vi "Get Segment Limits.vi"(8 "error in (no error)":errorcluster, 10 "segmentIdxIn":i32, 11 "TreeNode in":refnum<class "TreeNode.lvclass">) -> (0 "error out":errorcluster, 1 "End Data out":refnum<class "Data.lvclass">, 2 "Start Data out":refnum<class "Data.lvclass">, 3 "TreeNode out":refnum<class "TreeNode.lvclass">)   [LabVIEW 2012, in "MDSplus.lvlib" / "TreeNode.lvclass"]
uses:
  <vilib>/MDSplus/Classes/Data_Class/TreeNode_Class/TreeNode.lvclass
  <vilib>/MDSplus/Classes/Data_Class/Data.lvclass
  MDSobjectsLVShr.dll
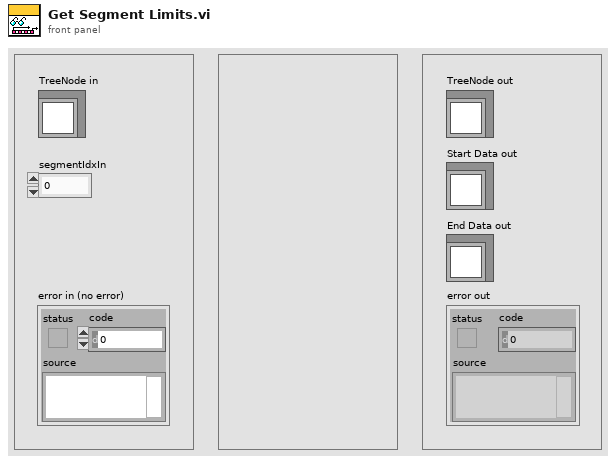
[diagram p1: front panel]
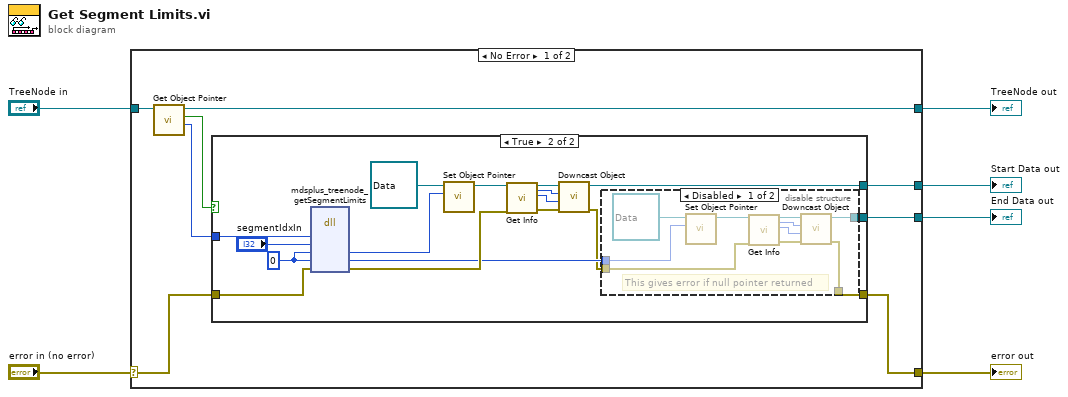
[diagram p0: block diagram]
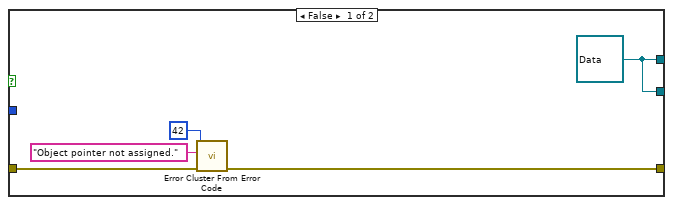
[diagram p2: hidden frame]
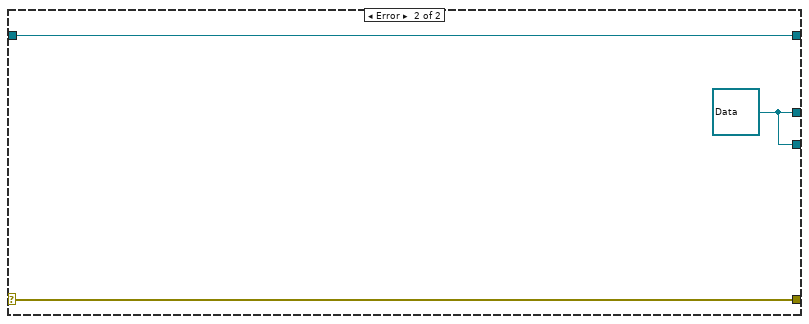
[diagram p4: hidden frame]
diagram:
  n1 = case shown="No Error" "error in (no error)" {
    selector: "error in (no error)" -> [w10 w50]
    tunnel: [w7 w50] -> w5
    tunnel: [w11 w49] -> w3
    tunnel: "TreeNode in" -> [w12 w49]
    tunnel: [w9 w48] -> w2
    tunnel: [w8 w48] -> w1
    frame No Error {
      n2 = call-dynamic "Get Object Pointer.vi"("Data in"=w12) -> ("Object Pointer"=w13:i64, "Assigned object pointer?"=w14:bool, "Data out"=w11:refnum<class "TreeNode.lvclass">)  [unwired: 8 in]
      n3 = case shown="True" w14 {
        tunnel: w13 -> [_ w36]
        tunnel: w10 -> [w17 w35]
        tunnel: [w16 w22] -> w7
        tunnel: [w15 w25] -> w9
        tunnel: [w15 w21] -> w8
        frame False {
          w15 = refnum<class "Data.lvclass"> refnum ("Data out")
          n4 = call <vilib>:"Error Cluster From Error Code.vi"("error in (no error)"=w17, "error message (\"\")"="Object pointer not assigned." ("error message (\"\")"), "error code (0)"=42) -> ("error out"=w16:errorcluster)  [unwired: 6 in]
        }
        frame True {
          w34 = i64 0 ("lvStartDataPtrOut")
          n5 = dll-call lib="MDSobjectsLVShr.dll" fn="mdsplus_treenode_getSegmentLimits"("lvTreeNodePtr"=w36, "segmentIdxIn"="segmentIdxIn", "lvStartDataPtrOut"=w34, "lvEndDataPtrOut"=w34, "error"=w35) -> ("lvStartDataPtrOut"=w27:i64, "lvEndDataPtrOut"=w24:i64, "error"=w26:errorcluster)  [unwired: 6 in, 2 out]
          n6 = call-dynamic "Set Object Pointer.vi"("Object Pointer"=w27, "Data in"=refnum<class "Data.lvclass"> refnum ("Data.lvclass")) -> ("Data out"=w32:refnum<class "Data.lvclass">)  [unwired: 9 in]
          n7 = call-dynamic "Get Info.vi"("Data in"=w32, "error in (no error)"=w26) -> ("Data out"=w31:refnum<class "Data.lvclass">, "Class type out"=w30:u8, "Data type out"=w29:u8, "error out"=w28:errorcluster)  [unwired: 12 in, 2 out]
          n8 = call <vilib>:"Downcast Object.vi"("error in (no error)"=w28, "Data Type"=w29, "Class Type"=w30, "Data in"=w31) -> ("error out"=w23:errorcluster, "Data out"=w25:refnum<class "Data.lvclass">)  [unwired: 6 in]
          n9 = disable-structure shown="Disabled" {
            disable-tunnel: w24 -> [w40 _]
            disable-tunnel: w23 -> [w39 w47]
            disable-tunnel: [w38 w47] -> w22
            disable-tunnel: [w37 _] -> w21
            frame Disabled {
              # "This gives error if null pointer returned"
              n10 = call-dynamic "Set Object Pointer.vi"("Object Pointer"=w40, "Data in"=refnum<class "Data.lvclass"> refnum ("Data.lvclass")) -> ("Data out"=w45:refnum<class "Data.lvclass">)  [unwired: 9 in]
              n11 = call-dynamic "Get Info.vi"("Data in"=w45, "error in (no error)"=w39) -> ("Data out"=w44:refnum<class "Data.lvclass">, "Class type out"=w43:u8, "Data type out"=w42:u8, "error out"=w41:errorcluster)  [unwired: 12 in, 2 out]
              n12 = call <vilib>:"Downcast Object.vi"("error in (no error)"=w41, "Data Type"=w42, "Class Type"=w43, "Data in"=w44) -> ("error out"=w38:errorcluster, "Data out"=w37:refnum<class "Data.lvclass">)  [unwired: 6 in]
            }
            frame Enabled {
            }
          }
        }
      }
    }
    frame Error {
      w48 = refnum<class "Data.lvclass"> refnum ("Data out")
    }
  }
  "error out" <- w5
  "TreeNode out" <- w3
  "Start Data out" <- w2
  "End Data out" <- w1
